vi "Write OVL Text.vi"(8 "error in (no error)":errorcluster, 10 "OVL Text":string, 11 "Static Text Overlay in":refnum<class "Static Text Overlay.lvclass">) -> (0 "error out":errorcluster, 3 "Static Text Overlay out":refnum<class "Static Text Overlay.lvclass">)   [LabVIEW 2014, in "Static Text Overlay.lvclass"]
uses:
  Static Text Overlay.lvclass
  Static Text Overlay.lvclass/Static Text Overlay.ctl
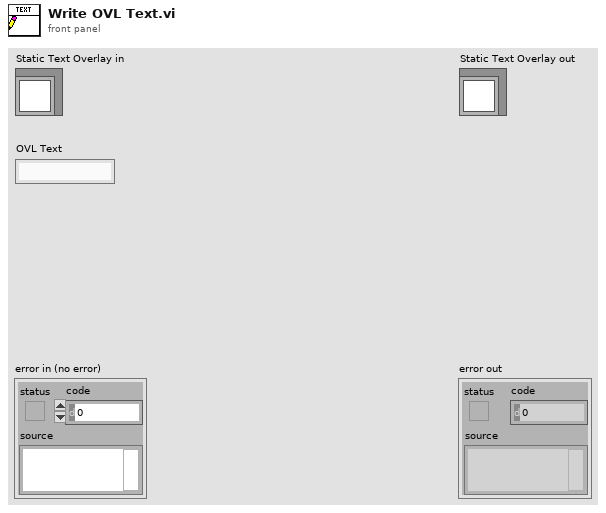
[diagram p1: front panel]
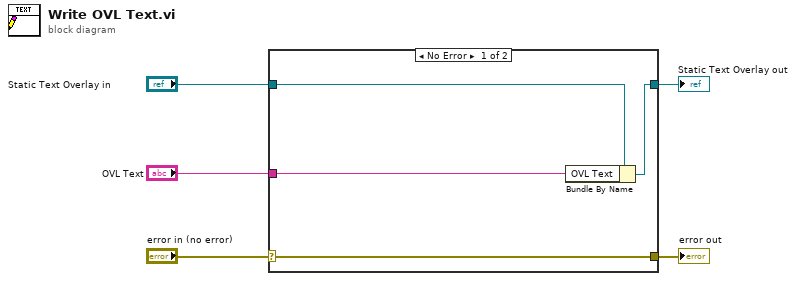
[diagram p0: block diagram]
diagram:
  n1 = case shown="No Error" "error in (no error)" {
    selector: "error in (no error)" -> [w9 w10]
    tunnel: [w9 w10] -> w4
    tunnel: [w7 w11] -> w2
    tunnel: "Static Text Overlay in" -> [w8 w11]
    tunnel: "OVL Text" -> [w6 _]
    frame No Error {
      n2 = Bundle By Name(cluster=w8, "OVL Text"=w6) -> (w7:refnum<class "Static Text Overlay.lvclass">)
    }
    frame Error {
    }
  }
  "error out" <- w4
  "Static Text Overlay out" <- w2
